vi "Convert Row Column to Address.vi"(8 "error in (no error)":errorcluster, 10 "cursor position":cluster{"row":i8, "column":i8} {"column" format="%.0x"}, 11 "cluster of private data in":T1={"FPGA VI Reference"=refnum, "device index"=0, "screen size"=enum."8x1", "font size"=enum."5x8", "auto wrap"=FALSE, "alignment"=enum."None", "number of line"=enum."2 lines", "shift 0"=0, "entry mode 0"=enum."increment & no shift", "shift 1"=0, "entry mode 1"=enum."increment & no shift"}) -> (0 "error out":errorcluster, 1 "address":u8, 3 "cluster of private data out":T1={"FPGA VI Reference"=refnum, "device index"=0, "screen size"=enum."8x1", "font size"=enum."5x8", "auto wrap"=FALSE, "alignment"=enum."None", "number of line"=enum."2 lines", "shift 0"=0, "entry mode 0"=enum."increment & no shift", "shift 1"=0, "entry mode 1"=enum."increment & no shift"}, 4 "chip select":enum16{"1st chip", "2nd chip"}(ring))   [LabVIEW 2017, in "HD44780.lvclass"]
uses:
  HD44780.lvclass
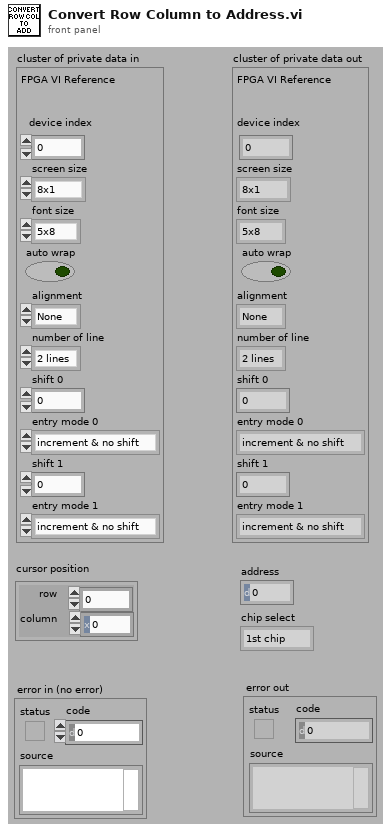
[diagram p1: front panel]
types:
  T1 = cluster{"FPGA VI Reference":refnum<k20>, "device index":i8, "screen size":enum8{"8x1", "8x2", "12x4", "16x1", "16x2", "16x4", "20x1", "20x2", "20x4", "24x1", "24x2", "40x2", "40x4"}, "font size":enum8{"5x8", "5x10"}, "auto wrap":bool, "alignment":enum16{"None", "Left", "Center", "Right"}, "number of line":enum8{"1 line", "2 lines"}, "shift 0":i8, "entry mode 0":enum8{"increment & no shift", "increment & shift", "decrement & no shift", "decrement & shift"}, "shift 1":i8, "entry mode 1":enum8{"increment & no shift", "increment & shift", "decrement & no shift", "decrement & shift"}}
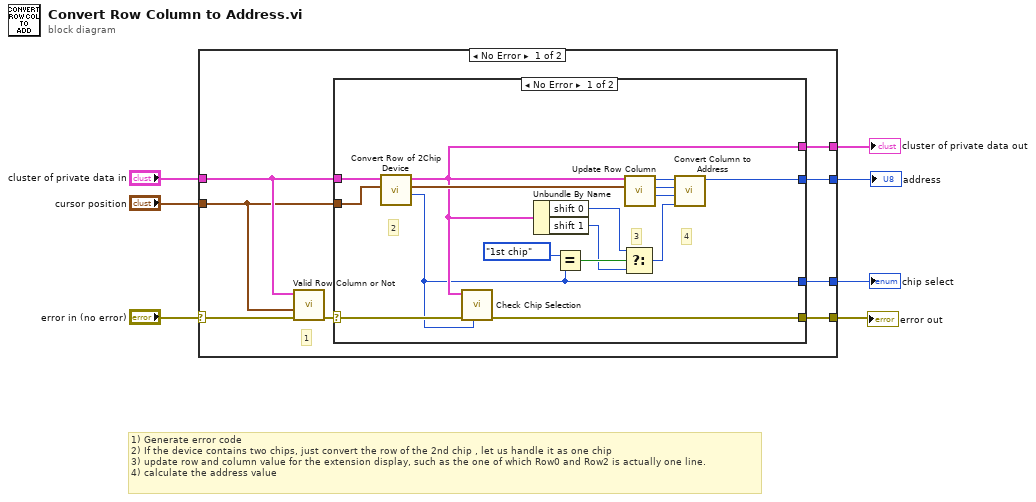
[diagram p0: block diagram]
diagram:
  # "1) Generate error code\n2) If the device contains two chips, just convert the row of the 2nd chip , let us handle it as one chip\n3) update row and column value for the extension display, such as the one of which Row0 and Row2 is actually one line.\n4) calculate the address value"
  n1 = case shown="No Error" "error in (no error)" {
    selector: "error in (no error)" -> [w10 w34]
    tunnel: [w14 w34] -> w7
    tunnel: "cursor position" -> [w8 _]
    tunnel: "cluster of private data in" -> [w9 w35]
    tunnel: [w13 w35] -> w4
    tunnel: [w12 _] -> w3
    tunnel: [w11 _] -> w2
    frame No Error {
      # "1"
      n2 = call "Valid Row Column or Not.vi"("error in (no error)"=w10, "cursor position in"=w8, "cluster of private data in"=w9) -> ("error out"=w15:errorcluster)  [unwired: 6 in, 2 out]
      n3 = case shown="No Error" w15 {
        selector: w15 -> [w19 w33]
        tunnel: [w17 w33] -> w14
        tunnel: w8 -> [w31 _]
        tunnel: w9 -> [w22 w32]
        tunnel: [w18 w32] -> w13
        tunnel: [w21 _] -> w12
        tunnel: [w16 _] -> w11
        frame No Error {
          # "4"
          # "3"
          # "2"
          n4 = call "Convert Row of 2Chip Device.vi"("cursor position"=w31, "cluster of private data in"=w22) -> ("chip select"=w16:enum16{"1st chip", "2nd chip"}, "current cursor position"=w30:cluster{"row":i8, "column":i8}, "cluster of private data output"=w18:T1)  [unwired: 7 in]
          n5 = call "Check Chip Selection.vi"("chip select"=w16, "error in (no error)"=w19, "cluster of private data in"=w18) -> ("error out"=w17:errorcluster)  [unwired: 7 in, 1 out]
          n6 = Unbundle By Name(w18) -> ("shift 0"=w25:i8, "shift 1"=w24:i8)
          n7 = Equal?(x=enum16{"1st chip", "2nd chip"}."1st chip" ("chip select 2"), y=w16) -> (x = y?=w29:bool)
          n8 = Select(t=w25, s=w29, f=w24) -> (s? t:f=w28:i8)
          n9 = call "Update Row Column.vi"("cursor position"=w30, "cluster of private data"=w18) -> ("max address"=w27:u8, "updated column"=w23:u8, "address of column zero"=w26:u8)  [unwired: 7 in]
          n10 = call "Convert Column to Address.vi"("shift value"=w28, "max address"=w27, "column(updated)"=w23, "address of column zero"=w26) -> ("address"=w21:u8)  [unwired: 7 in]
        }
        frame Error {
        }
      }
    }
    frame Error {
    }
  }
  "error out" <- w7
  "cluster of private data out" <- w4
  "address" <- w3
  "chip select" <- w2
